vi "Acquire.vi"(8 "error in (no error)":errorcluster, 10 "Msg in":T1, 11 "FakeCamera in":refnum<class "MoveDataFile.lvclass">) -> (0 "error out":errorcluster, 1 "new command":string, 2 "Msg out":T1, 3 "FakeCamera out":refnum<class "MoveDataFile.lvclass">)   [LabVIEW 2011, in "MoveDataFile.lvclass"]
uses:
  MoveDataFile.lvclass
  BaseDriver/DriverMsg.ctl
  shared/OnOffTypeDef.ctl
  MoveDataFile.lvclass/MoveDataFile.ctl
  shared/CompressAndUpdate(Poly)/CompressAndUpdate(Enum).vi
  BaseDriver/BaseDriver.lvclass
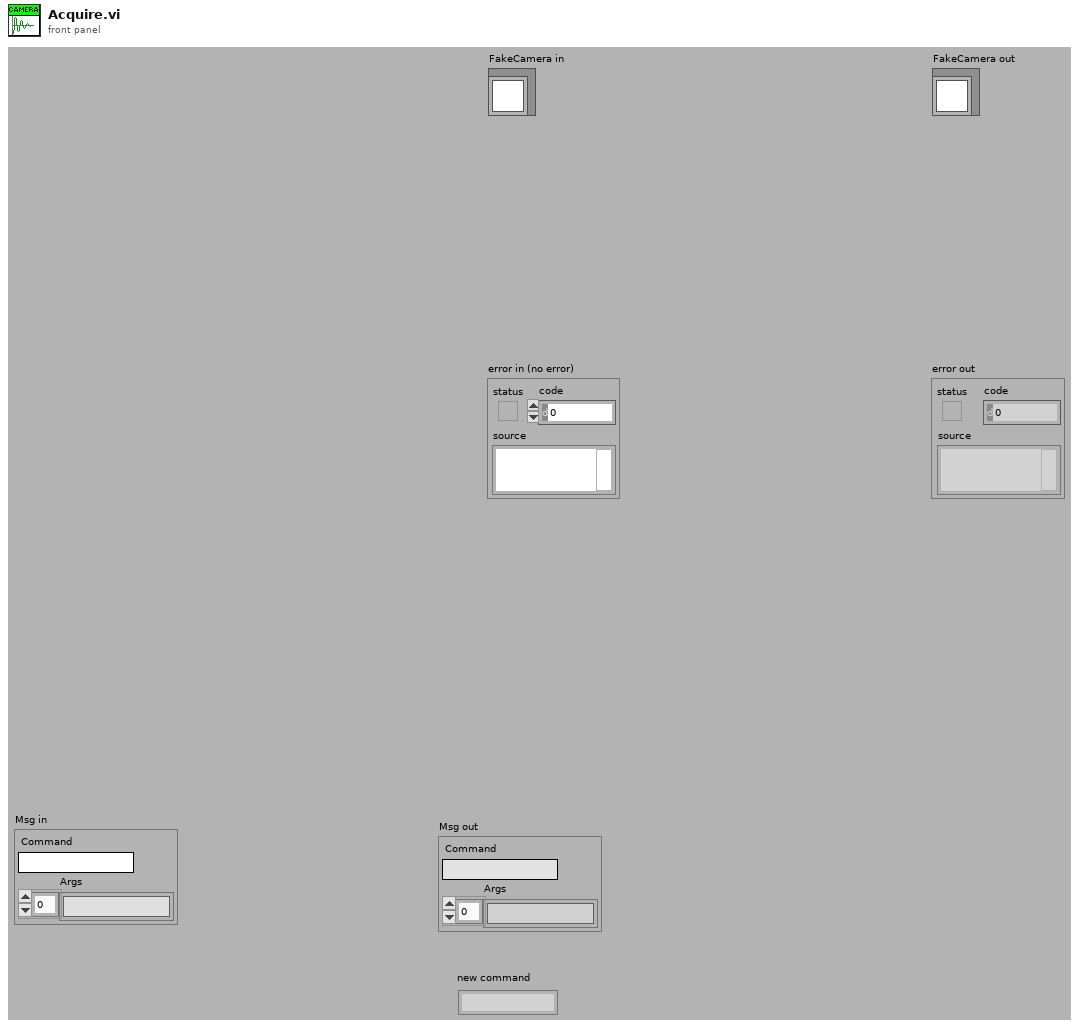
[diagram p1: front panel]
types:
  T1 = typedef "DriverMsg.ctl" = cluster{"Command":string, "Args":string[]}
  T2 = typedef "OnOffTypeDef.ctl" = enum16{"off", "on"}
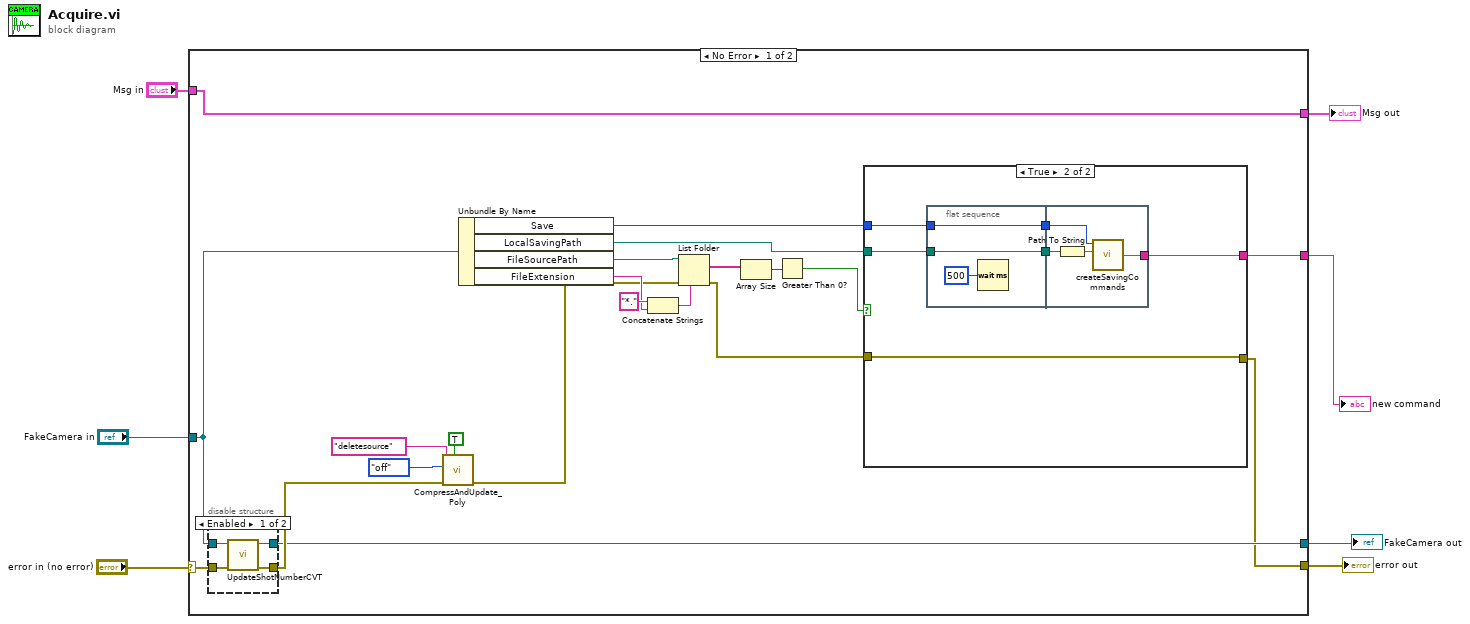
[diagram p0: block diagram]
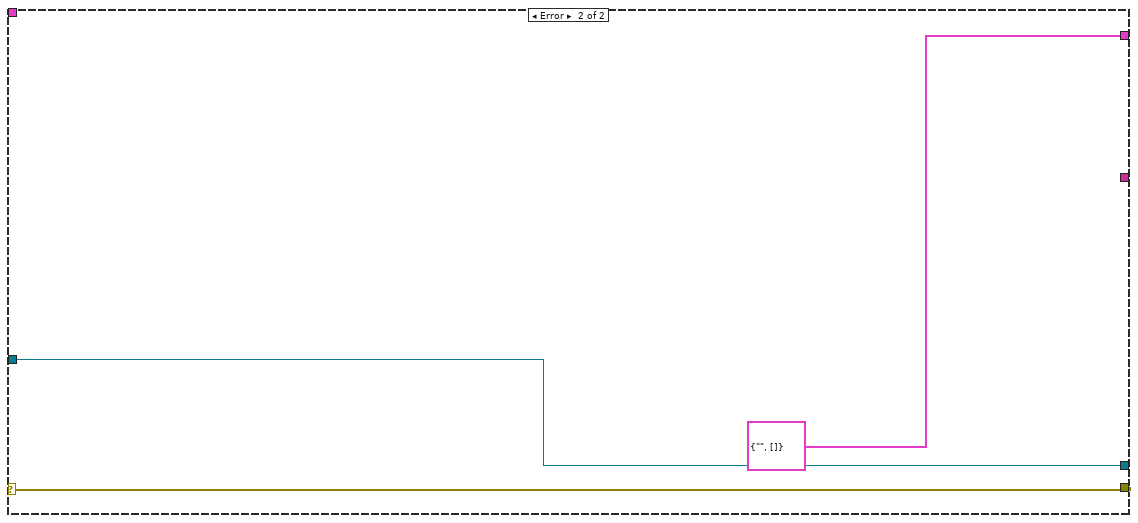
[diagram p4: hidden frame]
diagram:
  n1 = case shown="No Error" "error in (no error)" {
    selector: "error in (no error)" -> [w27 w51]
    tunnel: [w8 w51] -> w7
    tunnel: [w23 T1 {"Command"="", "Args"=[]} ("Msg out")] -> w2
    tunnel: [w11 w50] -> w6
    tunnel: "Msg in" -> [w23 _]
    tunnel: "FakeCamera in" -> [w28 w50]
    tunnel: [w12 _] -> w1
    frame No Error {
      n2 = disable-structure shown="Enabled" {
        disable-tunnel: w28 -> [w46 w48]
        disable-tunnel: [w45 w48] -> w11
        disable-tunnel: w27 -> [w44 w47]
        disable-tunnel: [w43 w47] -> w22
        frame Enabled {
          n3 = call "UpdateShotNumberCVT.vi"("error in (no error)"=w44, "BaseDriver in"=w46) -> ("error out"=w43:errorcluster, "BaseDriver out"=w45:refnum<class "MoveDataFile.lvclass">)  [unwired: 8 in]
        }
        frame Disabled {
        }
      }
      n4 = call-poly "CompressAndUpdate_Poly.vi"("force CVT update (false)"=TRUE ("force CVT update"), "error in"=w22, "enum variant"=OnOffTypeDef."off" ("Settings.Trigger"), "command or variable name"="deletesource") -> ("error out"=w18:errorcluster)  [unwired: 7 in]
      n5 = Unbundle By Name(w28) -> ("Save"=w14:T2, "LocalSavingPath"=w13:path, "FileSourcePath"=w17:path, "FileExtension"=w20:string)
      n6 = Concatenate Strings("*." ("string"), w20) -> (w19:string)
      n7 = List Folder(path=w17, pattern=w19, error in=w18) -> (filenames=w16:string[], error out=w9:errorcluster)  [unwired: 1 in, 2 out]
      n8 = Array Size(array=w16) -> (size(s)=w15:i32)
      n9 = Greater Than 0?(x=w15) -> (x > 0?=w10:bool)
      n10 = case shown="True" w10 {
        tunnel: w14 -> [_ w35]
        tunnel: w13 -> [_ w34]
        tunnel: [_ w33] -> w12
        tunnel: w9 -> [w29 w32]
        tunnel: [w29 w32] -> w8
        frame False {
        }
        frame True {
          n11 = flat-sequence {
            tunnel: w34 -> [w37]
            tunnel: w35 -> [w38]
            tunnel: [w38] -> w31
            tunnel: [w37] -> w30
            tunnel: [w39] -> w33
            tunnel: w31 -> [w42]
            tunnel: w30 -> [w41]
            frame #0 {
              n12 = Wait (ms)(milliseconds to wait=u32 500 ("millisecond multiple")) -> ()  [unwired: 1 out]
            }
            frame #1 {
              n13 = Path To String(path=w41) -> (string=w40:string)
              n14 = call "createSavingCommands.vi"("Saving Path (local)"=w40, "Save"=w42) -> ("String"=w39:string)  [unwired: 2 in]
            }
          }
        }
      }
    }
    frame Error {
    }
  }
  "error out" <- w7
  "FakeCamera out" <- w6
  "new command" <- w1
  "Msg out" <- w2
